vi "Make_Mirror_Pattern_V1.vi"(0 "Mirror Modes In":T1, 2 "Flat On?":bool, 7 "Flat File In":dbl[](array[numeric]), 11 "Mirror Modes Array":dbl[][](array[numeric])) -> (8 "Pixel Value U (-1 to 1)":dbl[](array[numeric]))   [LabVIEW 2014]
uses:
  Controls/MirrorModes.ctl
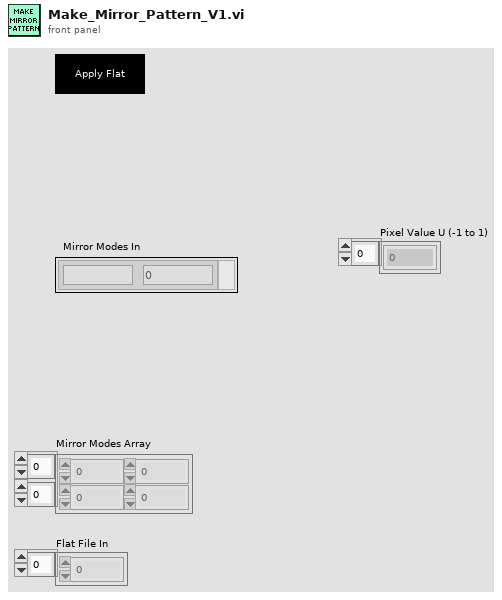
[diagram p1: front panel]
types:
  T1 = typedef "MirrorModes.ctl" = cluster{"Mode":string, "Amplitude":dbl}[]
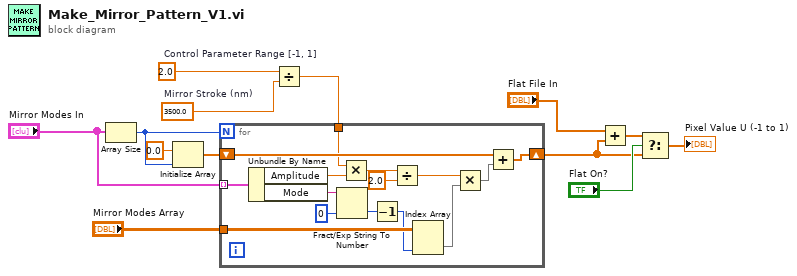
[diagram p0: block diagram]
diagram:
  w11 = 3500.0  # Mirror Stroke (nm)
  w10 = 2.0  # Control Parameter Range [-1, 1]
  n1 = Array Size(array="Mirror Modes In") -> (size(s)=w12:i32)
  n2 = Initialize Array(0.0 ("element"), w12) -> (w2:dbl[])
  n3 = Divide(x=w10, y=w11) -> (x/y=w9:dbl)
  n4 = for {
    N: w12 -> [_]
    tunnel: "Mirror Modes In" -> [w28] mode=indexing
    shift-right: [w21] -> w3
    shift-left: w2 -> [w22]
    tunnel: "Mirror Modes Array" -> [w24]
    tunnel: w9 -> [w15]
    n5 = Unbundle By Name(w28) -> ("Amplitude"=w16:dbl, "Mode"=w26:string)
    n6 = Fract/Exp String To Number(string=w26, default (0 dbl)=0) -> (number=w25:i32)  [unwired: 2 in, 1 out]
    n7 = Multiply(x=w15, y=w16) -> (x*y=w18:dbl)
    n8 = Decrement(x=w25) -> (x-1=w23:i32)
    n9 = Divide(x=w18, y=2.0) -> (x/y=w17:dbl)
    n10 = Index Array(array=w24, index (col)=w23) -> (element=w14:dbl[])  [unwired: 1 in]
    n11 = Multiply(x=w17, y=w14) -> (x*y=w20:dbl[])
    n12 = Add(x=w22, y=w20) -> (x+y=w21:dbl[])
  }
  n13 = Add(x="Flat File In", y=w3) -> (x+y=w8:dbl[])
  n14 = Select(t=w8, s="Flat On?", f=w3) -> (s? t:f=→"Pixel Value U (-1 to 1)":dbl[])
